vi "Transceiver Thread.Set Channels Buffer.vi"(10 "channels buffer":dbl[](array[numeric]), 11 "Transceiver Thread in":refnum<class "Transceiver Thread.lvclass">) -> (3 "Transceiver Thread out":refnum<class "Transceiver Thread.lvclass">)   [LabVIEW 2017, in "DSF Core.lvlib" / "Transceiver Thread.lvclass"]
uses:
  Transceiver Thread.lvclass
  Transceiver Thread.lvclass/Transceiver Thread.ctl
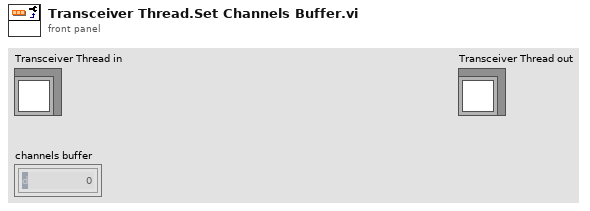
[diagram p1: front panel]
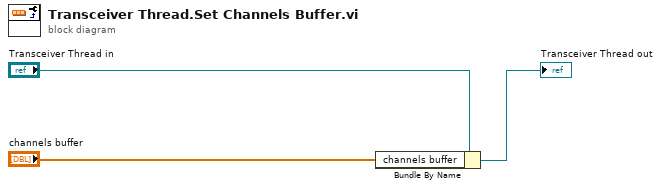
[diagram p0: block diagram]
diagram:
  n1 = Bundle By Name(cluster="Transceiver Thread in", "channels buffer"="channels buffer") -> (→"Transceiver Thread out":refnum<class "Transceiver Thread.lvclass">)
